vi "inittruser.vi"() -> ()   [LabVIEW 2014]
panel:
  out "Control Index 2":i32
  out "Control Index":i32
  in  "Array":string[][](array[string])
  in  "Write/Read":u16(ring) items=["Write", "Read"]
  in  "Numeric 7":u32
  in  "Numeric 6":i64
  in  "Numeric 5":dbl
  in  "Numeric 4":sgl
  in  "Numeric 3":u32
  in  "Numeric 2":i64
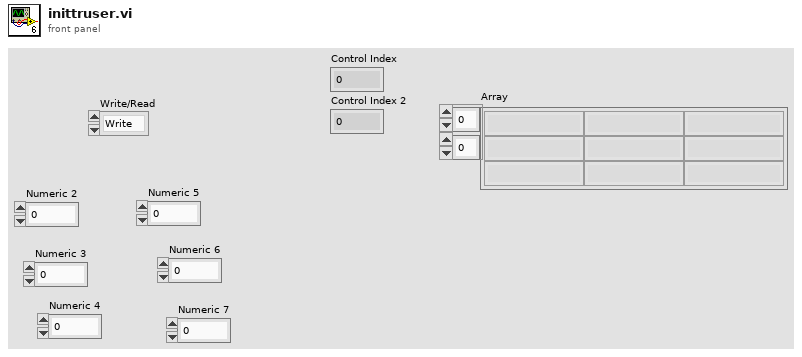
[diagram p1: front panel]
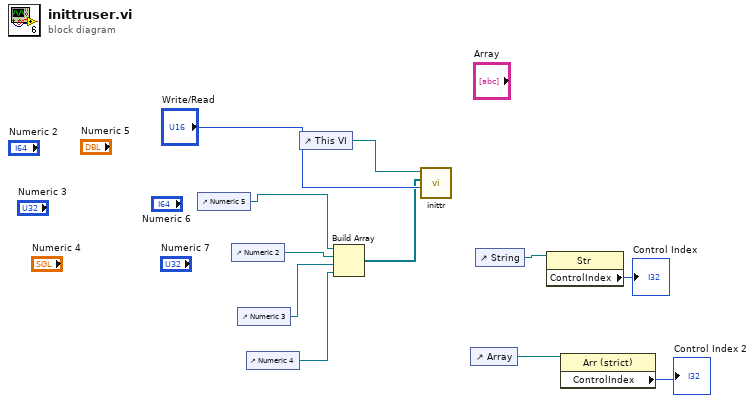
[diagram p0: block diagram]
diagram:
  n1 = control-ref of="Numeric 5"() -> (w8:refnum<vi>)
  n2 = control-ref of="Numeric 2"() -> (w11:refnum<vi>)
  n3 = control-ref of="Numeric 3"() -> (w10:refnum<vi>)
  n4 = control-ref of="Numeric 4"() -> (w9:refnum<vi>)
  n5 = control-ref of="This VI"() -> (w6:refnum<vi>)
  n6 = Build Array(w8, w11, w10, w9) -> (w5:refnum<vi>[])
  n7 = call "inittr.vi"("Write/Read"="Write/Read", "CtlRefs"=w5, 11:w6) -> ()  [unwired: 9 in]
  n8 = control-ref of="Array"() -> (w3:refnum<vi>)
  n9 = control-ref of="String"() -> (w4:refnum<vi>)
  n10 = property class="Str"(reference=w4) -> ("ControlIndex"=→"Control Index":i32)  [unwired: 1 in, 2 out]
  n11 = property class="Arr (strict)"(reference=w3) -> ("ControlIndex"=→"Control Index 2":i32)  [unwired: 1 in, 2 out]
